vi "mro_write_cmd.vi"(8 "error in (no error)":errorcluster, 10 "command":dbl[](array[numeric]), 11 "status in":i32) -> (0 "error out":errorcluster, 2 "return type":i8, 3 "status out":i32)   [LabVIEW 2011]
uses:
  mirao52e.dll
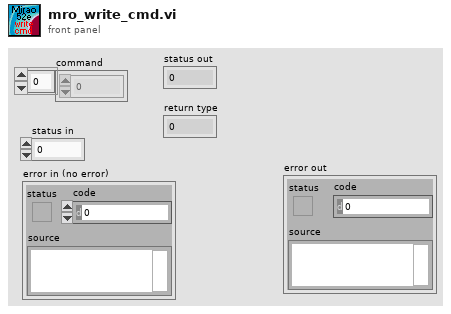
[diagram p1: front panel]
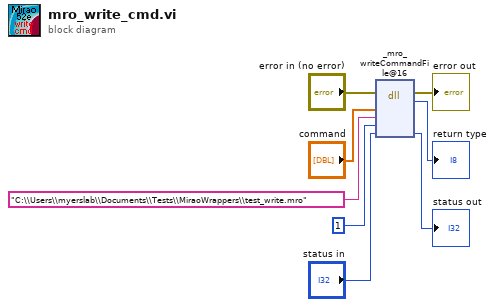
[diagram p0: block diagram]
diagram:
  n1 = dll-call lib="C:/Users/myerslab/workspace2/Mirao52J/labview/mirao52e.dll" fn="_mro_writeCommandFile@16"(error in="error in (no error)", "command"="command", "FilePath"="C:\\Users\\myerslab\\Documents\\Tests\\MiraoWrappers\\test_write.mro", "Overwrite"=1 ("trig"), "status"="status in") -> (error out=→"error out":errorcluster, "return type"=→"return type":i8, "status"=→"status out":i32)  [unwired: 5 in, 1 out]
